vi "Remote APIs for base station configuration SET.vi"(1 "Cellular Technology":T3, 2 "Base Station":T2, 3 "Heading":T1, 4 "Sub-Heading":string, 5 "Value":string, 7 "error in (no error)":errorcluster) -> (27 "error out":errorcluster)   [LabVIEW 2021]
uses:
  Controls/TCP_FGV.ctl
  Controls/Base_Station_Emulator.ctl
  Controls/Cellular_Technology.ctl
  Set,Get_Configuration_Controls/Heading.ctl
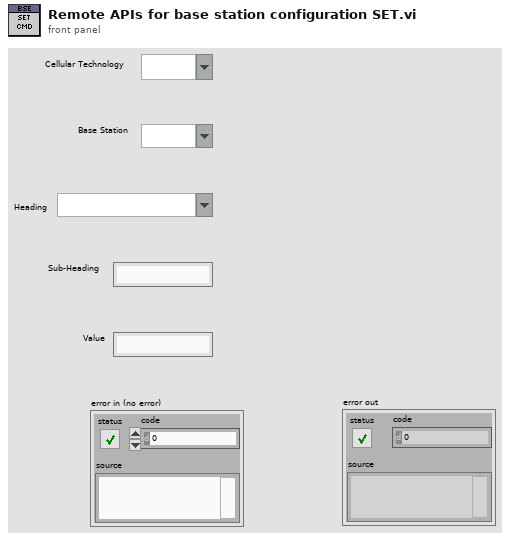
[diagram p1: front panel]
types:
  T1 = typedef "Heading.ctl" = string
  T2 = typedef "Base_Station_Emulator.ctl" = string
  T3 = typedef "Cellular_Technology.ctl" = string
  T4 = typedef "TCP_FGV.ctl" = enum16{"Open", "Read", "Write", "Close"}
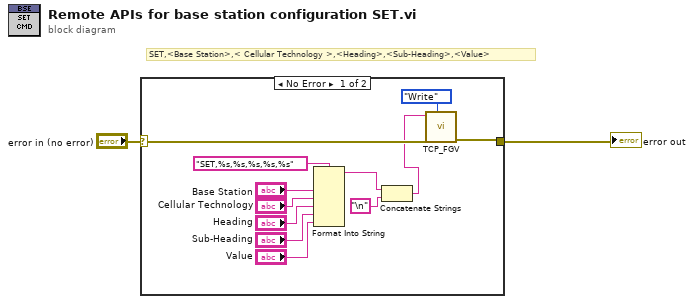
[diagram p0: block diagram]
diagram:
  # "SET,<Base Station>,< Cellular Technology >,<Heading>,<Sub-Heading>,<Value>"
  n1 = case shown="No Error" "error in (no error)" {
    selector: "error in (no error)" -> [w7 w15]
    tunnel: [w8 w15] -> w2
    frame No Error {
      n2 = Format Into String(format string="SET,%s,%s,%s,%s,%s", "Base Station", "Cellular Technology", "Heading", "Sub-Heading", "Value") -> (resulting string=w4:string)  [unwired: 2 in, 1 out]
      n3 = Concatenate Strings(w4, "\n") -> (w3:string)
      n4 = call "TCP_FGV.vi"("Command"=w3, "error in (no error)"=w7, "Operation"=TCP_FGV."Write") -> ("error out"=w8:errorcluster)  [unwired: 6 in, 1 out]
    }
    frame Error {
    }
  }
  "error out" <- w2
